vi "원그리기.vi"() -> ()   [LabVIEW 2014]
uses:
  <vilib>/Analysis/NI_AALBase.lvlib
panel:
  out "XY 그래프":cluster{"sine wave":dbl[], "sine wave":dbl[]}[](graph)
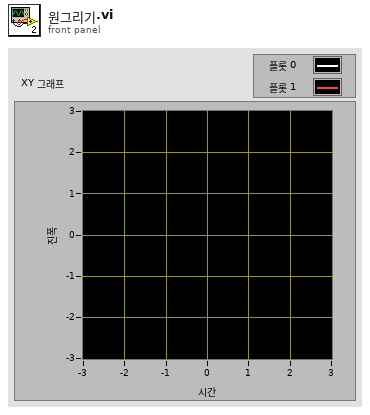
[diagram p1: front panel]
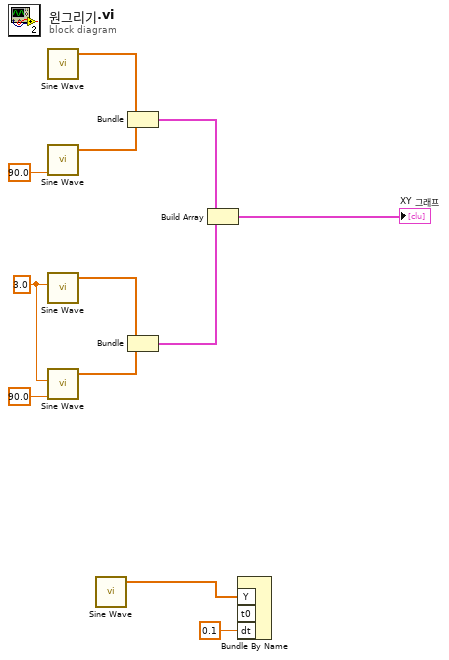
[diagram p0: block diagram]
diagram:
  w4 = 3.0 ("amplitude")
  n1 = call <vilib>:"Sine Wave.vi"() -> ("sine wave"=w12:dbl[])  [unwired: 5 in, 2 out]
  n2 = call <vilib>:"Sine Wave.vi"("phase in"=90.0) -> ("sine wave"=w11:dbl[])  [unwired: 4 in, 2 out]
  n3 = call <vilib>:"Sine Wave.vi"("amplitude"=w4) -> ("sine wave"=w7:dbl[])  [unwired: 4 in, 2 out]
  n4 = call <vilib>:"Sine Wave.vi"("amplitude"=w4, "phase in"=90.0) -> ("sine wave"=w8:dbl[])  [unwired: 3 in, 2 out]
  n5 = call <vilib>:"Sine Wave.vi"() -> ("sine wave"=w2:dbl[])  [unwired: 5 in, 2 out]
  n6 = Bundle("sine wave"=w12, "sine wave"=w11) -> (w6:cluster{"sine wave":dbl[], "sine wave":dbl[]})  [unwired: 1 in]
  n7 = Bundle("sine wave"=w7, "sine wave"=w8) -> (w5:cluster{"sine wave":dbl[], "sine wave":dbl[]})  [unwired: 1 in]
  n8 = Build Array(w6, w5) -> (→"XY 그래프":cluster{"sine wave":dbl[], "sine wave":dbl[]}[])
  n9 = Bundle By Name("Y"=w2, "dt"=0.1) -> ()  [unwired: 2 in, 1 out]
